vi "Update Results.vi"(8 "error in (no error)":errorcluster, 10 "Measurement Results":variant, 11 "MeasurementContext in":refnum<class "MeasurementContext.lvclass">) -> (0 "error out":errorcluster, 3 "MeasurementContext out":refnum<class "MeasurementContext.lvclass">)   [LabVIEW 2020, in "MeasurementLink Measurement Server.lvlib" / "MeasurementContext.lvclass"]
doc: "Sends measurement updates to a measurement client, like InstrumentStudio. Do not use this VI to write the final results. Instead, use the Measurement Results indicator of the Measurement Logic VI to write the final measurement result.\n\nThis VI must be called with the Measurement Results cluster as the input. You must always update all elements of the cluster, including unchanged values.\n\nInstrumentStudio does not cache data from previous updates so you must write all of the data to the cluster to display cumulative updates.\n\nTestStand gnores updates from this VI and only uses the final measurement result."
uses:
  MeasurementContext.lvclass
  IMeasurementService/IMeasurementService.lvclass
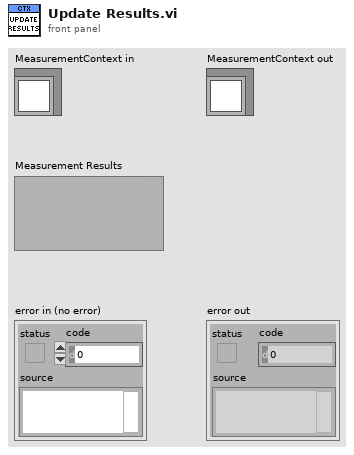
[diagram p1: front panel]
types:
  T1 = typedef "grpc-lvsupport-release.lvlib/grpcId.ctl" = u64
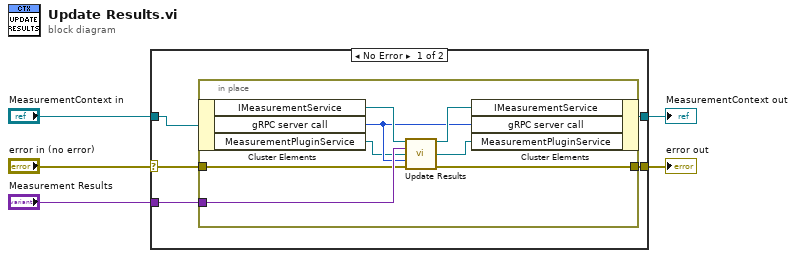
[diagram p0: block diagram]
diagram:
  n1 = case shown="No Error" "error in (no error)" {
    selector: "error in (no error)" -> [w8 w20]
    tunnel: [w7 w20] -> w4
    tunnel: [w6 w19] -> w2
    tunnel: "MeasurementContext in" -> [w10 w19]
    tunnel: "Measurement Results" -> [w9 _]
    frame No Error {
      n2 = in-place {
        in-place-border: w9 -> [w16]
        in-place-border: w8 -> [w15]
        in-place-border: [w14] -> w7
        n3 = in-place-cluster #1(w10) -> ("IMeasurementService"=w18:refnum<class "IMeasurementService.lvclass">, "gRPC server call"=w13:T1, "MeasurementPluginService"=w12:refnum<class "MeasurementPluginService.lvclass">)
        n4 = call-dynamic "Update Results.vi"("IMeasurementService in"=w18, "Measurement Results"=w16, "MeasurementPluginService in"=w12, "gRPCid in"=w13, "error in (no error)"=w15) -> ("IMeasurementService out"=w17:refnum<class "IMeasurementService.lvclass">, "MeasurementPluginService out"=w11:refnum<class "MeasurementPluginService.lvclass">, "error out"=w14:errorcluster)  [unwired: 8 in]
        n5 = in-place-cluster #1("IMeasurementService"=w17, "gRPC server call"=w13, "MeasurementPluginService"=w11) -> (w6:refnum<class "MeasurementContext.lvclass">)
      }
    }
    frame Error {
    }
  }
  "error out" <- w4
  "MeasurementContext out" <- w2
